vi "LuaVIEW Bootstrap.vi"(0 "script file or name (no name)":path, 5 "custom search directory (none)":path, 7 "script string (\"\" == load from file)":string, 9 "task alternatives (default)":refnum<vi>[](array[refnum]), 11 "error in (no error)":errorcluster) -> (15 "error out":errorcluster)   [LabVIEW 2012]
doc: "Bootstrap an application that uses LuaVIEW with a Lua script. Note that this VI is intentionally non-reentrant so that only a single bootstrap script can be active at any one time. The bootstrap script can set the global configuration and register functions prior to starting further Lua scripts. To do so, the bootstrap script has access to all C functions and a small set of LuaVIEW functions:\nconfigure(tab:configuration)\nstr:path=bootstrap_path()\nstr:path=toolkit_path(str:toolkit,[str:subpath])\nstr:kind=app_kind()\nregister.public(str:path)\nregister.public_dir(str:dirpath)\ndo_script(str:name,[str:script])\nThe last four are identical to the standard LuaVIEW functions of the same name. The configure() function is used to set the configuration globals. See the bootstrapping example VI for details. When the bootstrap script was loaded from a file instead of passed as a string, the bootstrap_path() function returns a path to the directory containing the script. This allows the resource base path or script search directories to be configured relative to this path.\n\nThough bootstrapping can also be done with LabVIEW code that sets configuration globals and calls the LabVIEW API to register functions, the advantages of a bootstrap script are that it has convenient error handling and can be changed when deployed with a built executable."
uses:
  private/LuaVIEW Push (path).vi
  private/LuaVIEW Push (string).vi
  private/LuaVIEW Push (flat data).vi
  private/LuaVIEW Push (refnum).vi
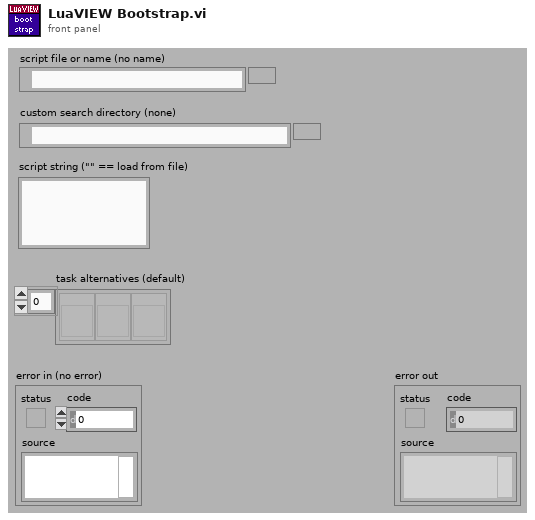
[diagram p1: front panel]
types:
  T1 = typedef "t_LuaVIEW Reference.ctl" = refnum<k1>
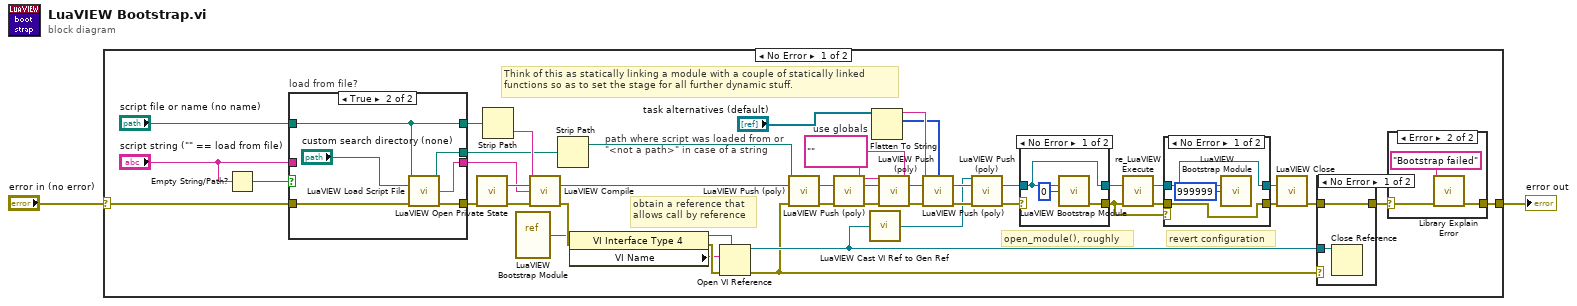
[diagram p0: block diagram]
diagram:
  n1 = case shown="No Error" "error in (no error)" {
    selector: "error in (no error)" -> [w37 w73]
    tunnel: [w4 w73] -> w2
    frame No Error {
      w27 = ""  # use globals
      # "path where script was loaded from or\n\"<not a path>\" in case of a string"
      # "Think of this as statically linking a module with a couple of statically linked\nfunctions so as to set the stage for all further dynamic stuff."
      # "revert configuration"
      # "open_module(), roughly"
      # "obtain a reference that\nallows call by reference"
      n2 = Empty String/Path?(string/path="script string (\"\" == load from file)") -> (empty?=w43:bool)
      n3 = case "load from file?" shown="True" w43 {
        tunnel: [w65 w72] -> w44
        tunnel: w37 -> [w65 w71]
        tunnel: "script string (\"\" == load from file)" -> [w66 _]
        tunnel: [w66 w70] -> w42
        tunnel: "script file or name (no name)" -> [w64 w69]
        tunnel: [w64 w69] -> w41
        tunnel: [_ w67] -> w20
        frame False {
        }
        frame True {
          n4 = call "LuaVIEW Load Script File.vi"("script file"=w69, "custom search directory (none)"="custom search directory (none)", "error in (no error)"=w71) -> ("absolute path"=w67:path, "script text"=w70:string, "error out"=w72:errorcluster)  [unwired: 8 in, 2 out]
        }
      }
      n5 = call "LuaVIEW Open Private State.vi"("error in (no error)"=w44) -> ("LuaVIEW reference"=w45:T1, "error out"=w46:errorcluster)  [unwired: 13 in]
      n6 = Strip Path(path=w41) -> (name=w40:string)  [unwired: 1 out]
      n7 = vi-ref "LuaVIEW Bootstrap Module.vi"() -> ("vi reference"=w26:refnum<vi>)
      n8 = call "LuaVIEW Compile.vi"("script name"=w40, "LuaVIEW reference in"=w45, "script"=w42, "error in (no error)"=w46) -> ("LuaVIEW reference out"=w16:T1, "error out"=w33:errorcluster)  [unwired: 10 in]
      n9 = Strip Path(path=w20) -> (stripped path=w17:path)  [unwired: 1 out]
      n10 = property class="VI Interface Type 4"(reference=w26, error in=w33) -> (reference out=w35:refnum<vi>, error out=w36:errorcluster, "VI Name"=w34:string)
      n11 = Open VI Reference(type specifier VI Refnum (for type only)=w35, vi path=w34, error in (no error)=w36) -> (vi reference=w30:refnum<vi>, error out=w15:errorcluster)  [unwired: 3 in]
      n12 = call-poly "LuaVIEW Push (poly).vi"("path"=w17, "LuaVIEW reference in"=w16, "error in (no error)"=w15) -> ("LuaVIEW reference out"=w18:T1, "error out"=w19:errorcluster)  [unwired: 11 in]
      n13 = call-poly "LuaVIEW Push (poly).vi"("string"=w27, "LuaVIEW reference in"=w18, "error in (no error)"=w19) -> ("LuaVIEW reference out"=w29:T1, "error out"=w28:errorcluster)  [unwired: 11 in]
      n14 = call "LuaVIEW Cast VI Ref to Gen Ref.vi"("refnum in"=w30) -> ("refnum out"=w5:refnum<vi>)  [unwired: 14 in]
      n15 = Flatten To String(anything="task alternatives (default)") -> (data string=w14:string, type string=w13:i16[])  [unwired: 3 in, 1 out]
      n16 = call-poly "LuaVIEW Push (poly).vi"("string"=w27, "LuaVIEW reference in"=w29, "error in (no error)"=w28) -> ("LuaVIEW reference out"=w11:T1, "error out"=w10:errorcluster)  [unwired: 11 in]
      n17 = call-poly "LuaVIEW Push (poly).vi"("flat data"=w14, "type descriptor"=w13, "LuaVIEW reference in"=w11, "error in (no error)"=w10) -> ("LuaVIEW reference out"=w6:T1, "error out"=w7:errorcluster)  [unwired: 10 in]
      n18 = call-poly "LuaVIEW Push (poly).vi"("refnum"=w5, "LuaVIEW reference in"=w6, "error in (no error)"=w7) -> ("LuaVIEW reference out"=w9:T1, "error out"=w8:errorcluster)  [unwired: 11 in]
      n19 = case shown="No Error" w8 {
        selector: w8 -> [_ w63]
        tunnel: [w61 w63] -> w22
        tunnel: w9 -> [w59 w62]
        tunnel: [w59 w62] -> w32
        frame No Error {
          n20 = call "LuaVIEW Bootstrap Module.vi"("LuaVIEW reference"=w59, "function index"=0) -> ("error out"=w61:errorcluster)  [unwired: 13 in]
        }
        frame Error {
        }
      }
      n21 = call "re_LuaVIEW Execute.vi"("LuaVIEW reference in"=w32, "error in (no error)"=w22) -> ("LuaVIEW reference out"=w25:T1, "error out"=w21:errorcluster)  [unwired: 12 in]
      n22 = case shown="No Error" w22 {
        selector: w22 -> [_ w55]
        tunnel: [w51 w55] -> w24
        tunnel: w25 -> [w52 w54]
        tunnel: [w52 w54] -> w23
        tunnel: w21 -> [w51 _]
        frame No Error {
          n23 = call "LuaVIEW Bootstrap Module.vi"("LuaVIEW reference"=w52, "function index"=999999) -> ()  [unwired: 13 in, 1 out]
        }
        frame Error {
        }
      }
      n24 = call "LuaVIEW Close.vi"("LuaVIEW reference"=w23, "error in (no error)"=w24) -> ("dup error"=w31:errorcluster)  [unwired: 13 in]
      n25 = case shown="No Error" w15 {
        tunnel: w31 -> [w56 w58]
        tunnel: w30 -> [w57 _]
        tunnel: [w56 w58] -> w3
        frame No Error {
          n26 = Close Reference(reference=w57) -> ()  [unwired: 1 in, 1 out]
        }
        frame Error {
        }
      }
      n27 = case shown="Error" w3 {
        selector: w3 -> [w47 w49]
        tunnel: [w47 w50] -> w4
        frame No Error {
        }
        frame Error {
          n28 = call "Library Explain Error.vi"("explanation prefix (none)"="Bootstrap failed", "error in (no error)"=w49) -> ("explained error"=w50:errorcluster)  [unwired: 13 in]
        }
      }
    }
    frame Error {
    }
  }
  "error out" <- w2
